vi "6.3.vi"() -> ()   [LabVIEW 2017]
uses:
  <vilib>/measure/NI_MABase.lvlib
panel:
  in  "路径":path
  in  "phase":dbl caption="相位" format="%.2p"
  in  "amplitude":dbl=1.0 caption="幅值" format="%0.2p"
  in  "frequency":dbl=10.0 caption="频率" format="%0.2p"
  out "Y":dbl[](array[numeric])
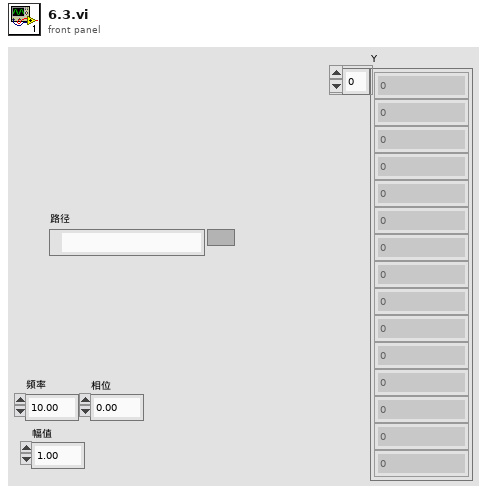
[diagram p1: front panel]
types:
  T1 = enum16{"open", "replace", "create", "open or create", "replace or create", "replace or create with confirmation"}
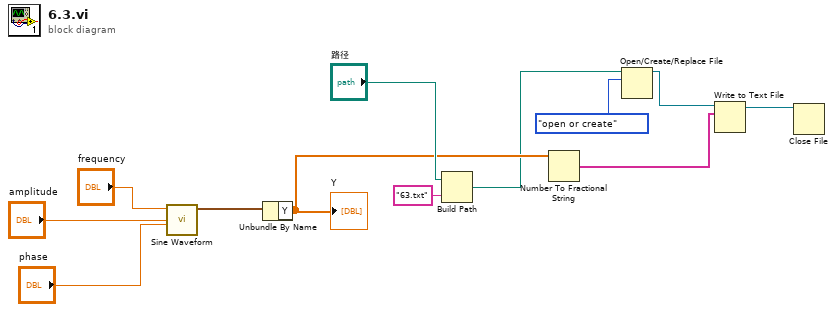
[diagram p0: block diagram]
diagram:
  n1 = call <vilib>:"Sine Waveform.vi"("phase"="phase", "amplitude"="amplitude", "frequency"="frequency") -> ("signal out"=w12:waveform(dbl))  [unwired: 7 in, 1 out]
  n2 = Unbundle By Name(w12) -> ("Y"=w5:dbl[])
  "Y" <- w5
  n3 = Build Path(base path="路径", name or relative path="63.txt" ("名称或相对路径")) -> (appended path=w3:path)
  n4 = Number To Fractional String(number=w5) -> (F-format string=w4:string[])  [unwired: 3 in]
  n5 = Open/Create/Replace File(file path (use dialog)=w3, operation (0:open)=T1."open or create" ("操作(0:open)")) -> (refnum out=w1:refnum<file>)  [unwired: 4 in, 2 out]
  n6 = Write to Text File(file (use dialog)=w1, text=w4) -> (refnum out=w6:refnum<file>)  [unwired: 2 in, 2 out]
  n7 = Close File(refnum=w6) -> ()  [unwired: 1 in, 2 out]
